vi "SERIAL_Write.vi"(8 "error in (no error)":errorcluster, 9 "Message":u8[](array[numeric]), 10 "Device Register":T2 items=["WHOAMI"=0, "HW_REV"=1, "FW_VER_MAJOR"=2, "FW_VER_MINOR"=3, "UPDATE_RATE_HZ"=4, "ACCEL_FSR_G"=5, "GYRO_FSR_DPS"=6, "OP_STATUS"=8, "CAL_STATUS"=9, "SELFTEST_STATUS"=10, "CAPABILITY_FLAGS_L"=11, "CAPABILITY_FLAGS_H"=12, "SENSOR_STATUS"=16, "TIMESTAMP"=18, "YAW"=22, "PITCH"=24, "ROLL"=26, "HEADING"=28, "FUSED_HEADING"=30, "ALTITUDE_I"=32, "ALTITUDE_D"=34, "LINERA_ACC_X"=36, "LINERA_ACC_Y"=38, "LINERA_ACC_Z"=40, "QUAT_W"=42, "QUAT_X"=44, "QUAT_Y"=46, "QUAT_Z"=48, "MPU_TEMP_C"=50, "GYRO_X"=52, "GYRO_Y"=54, "GYRO_Z"=56, "ACC_X"=58, "ACC_Y"=60, "ACC_Z"=62, "MAG_X"=64, "MAG_Y"=66, "MAG_Z"=68, "PRESSURE_I"=70, "PRESSURE_D"=72, "PRESSURE_TEMP"=74, "YAW_OFFSET"=76, "QUAT_OFFSET_W"=78, "QUAT_OFFSET_X"=80, "QUAT_OFFSET_Y"=82, "QUAT_OFFSET_Z"=84, "INTEGRATION_CONTROL"=86, "VELOCITY_X"=88, "VELOCITY_Y"=92, "VELOCITY_Z"=96, "DISPLACMENT_X"=100, "DISPLACMENT_Y"=104, "DISPLACEMENT_Z"=108], 11 "SerialPortRef":T1) -> (0 "error out":errorcluster, 3 "SerialPortRef":T1)   [LabVIEW 2014, in "navX-MXP IMU.lvlib"]
uses:
  navX-MXP IMU.lvlib
  COMMON/TypeDefs/Value TypeDefs/navX Device Registers.ctl
  <vilib>/Rock Robotics/WPI/SerialPort/WPI_SerialPortRef.ctl
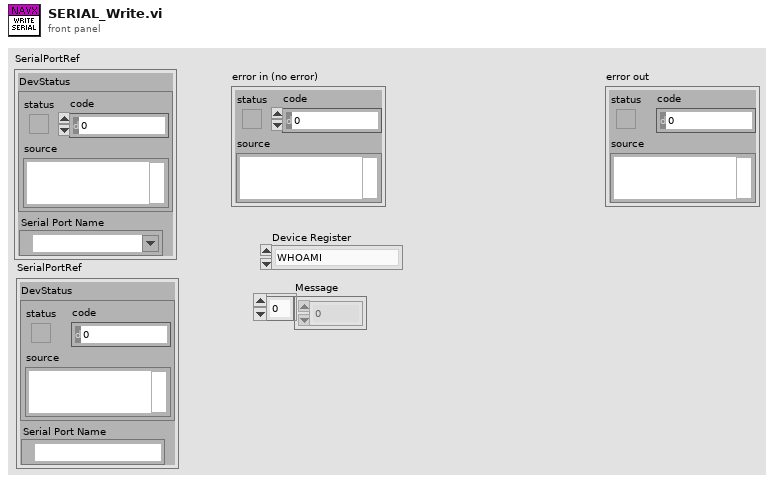
[diagram p1: front panel]
types:
  T1 = typedef "WPI_SerialPortRef.ctl" = cluster{"DevStatus":errorcluster, "Serial Port Name":refnum<visa-resource-name>}
  T2 = typedef "navX-MXP IMU.lvlib/navX Device Registers.ctl" = u8
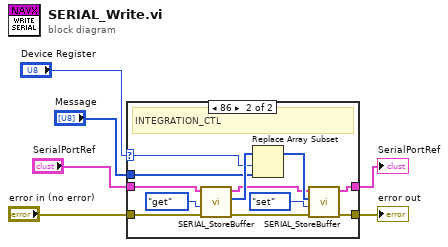
[diagram p0: block diagram]
diagram:
  n1 = case shown="86" "Device Register" {
    selector: "Device Register" -> [_ w13]
    tunnel: "Message" -> [_ w12]
    tunnel: [w8 w20] -> w4
    tunnel: "SerialPortRef" -> [w8 w16]
    tunnel: [w7 w19] -> w2
    tunnel: "error in (no error)" -> [w7 w15]
    frame Default {
    }
    frame 86 {
      # "INTEGRATION_CTL"
      n2 = call "SERIAL_StoreBuffer.vi"("error in (no error)"=w15, "Access Type"=enum16{"set", "get", "delete"}."get", "SerialPortRef"=w16) -> ("error out"=w9:errorcluster, "navX Data"=w14:u8[], "SerialPortRef"=w10:T1)  [unwired: 6 in]
      n3 = Replace Array Subset(array=w14, new element=w12, index=w13) -> (w11:u8[])
      n4 = call "SERIAL_StoreBuffer.vi"("error in (no error)"=w9, "Access Type"=enum16{"set", "get", "delete"}."set", "navX Data"=w11, "SerialPortRef"=w10) -> ("error out"=w19:errorcluster, "SerialPortRef"=w20:T1)  [unwired: 5 in, 1 out]
    }
  }
  "error out" <- w2
  "SerialPortRef" <- w4
